vi "UpdateClibWithNewB.vi"(8 "error in (no error)":errorcluster, 11 "MagSpec_Bella in":refnum<class "MagSpec_Bella.lvclass">) -> (0 "error out":errorcluster, 3 "MagSpec_Bella out":refnum<class "MagSpec_Bella.lvclass">)   [LabVIEW 2013, in "MagSpec_Bella.lvclass"]
uses:
  MagSpec_Bella.lvclass
  MagSpec_Bella.lvclass/MagSpec_Bella.ctl
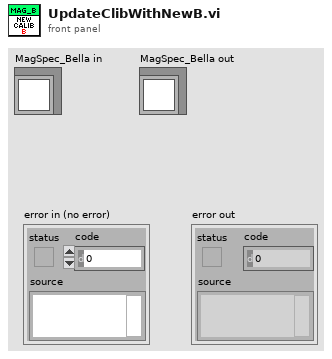
[diagram p1: front panel]
types:
  T1 = typedef "Calibration_Pixel_based.ctl" = cluster{"y1(pixel)":dbl[], "y2(pixel)":dbl[], "dp/B [MeV/C/B] (pixel)":dbl[], "energyDependence Input(pixel)":dbl[], "bending angle [deg](pixel)":dbl[], "total path(pixel)":dbl[], "pixel angle (y)(pixel)":dbl[], "energy dependence (pixel)":dbl[], "charge compensation (pixel)":dbl[], "Momentum [MeV/C](pixel)":dbl[], "angular compensation(pixel)":dbl[]}
  T2 = typedef "CameraSettings_File.ctl" = cluster{"FOV [mm]":dbl, "Left edge [mm]":dbl, "ROI Y offset":dbl, "ROI height":dbl, "ROI X offset":dbl, "ROI width":dbl, "Y center pixel":dbl, "Y Start":dbl, "Y End":dbl, "X Start":dbl, "X End":dbl, "rot [deg]":dbl}
  T3 = typedef "2D.ctl" = cluster{"dp":dbl[][], "chargeCompensation":dbl[][], "angle":dbl[][], "Momentum":dbl[][]}
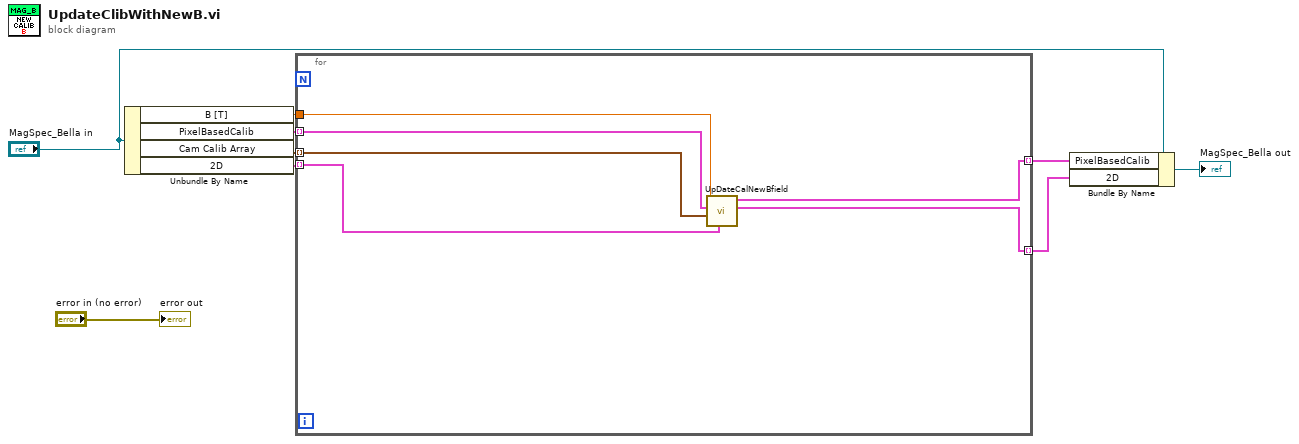
[diagram p0: block diagram]
diagram:
  n1 = Unbundle By Name("MagSpec_Bella in") -> ("B [T]"=w2:dbl, "PixelBasedCalib"=w6:T1[], "Cam Calib Array"=w4:T2[], "2D"=w1:T3[])
  n2 = for {
    tunnel: w6 -> [w15] mode=indexing
    tunnel: [w14] -> w8 mode=indexing
    tunnel: w2 -> [w13]
    tunnel: w1 -> [w11] mode=indexing
    tunnel: [w12] -> w5 mode=indexing
    tunnel: w4 -> [w10] mode=indexing
    n3 = call "UpDateCalNewBfield.vi"("2D in"=w11, "Camera Settings"=w10, "Cluster in"=w15, "B [T]"=w13) -> ("2D out"=w12:T3, "Cluster out"=w14:T1)  [unwired: 6 in]
  }
  n4 = Bundle By Name(cluster="MagSpec_Bella in", "PixelBasedCalib"=w8, "2D"=w5) -> (→"MagSpec_Bella out":refnum<class "MagSpec_Bella.lvclass">)
  "error out" <- "error in (no error)"
